vi "Mass Dependent Parameters.vi"(5 "Current Mass Range":i32(ring) items=["Mass Range 1"], 7 "Mass Ranges":T1[](array[typedef]) {"Res" items=["High/High", "Medium/Medium", "Low/Low", "High/Medium", "High/Low", "Medium/High", "Medium/Low", "Low/High", "Low/Medium"]}) -> (3 "Mass Ranges Out":T1[](array[typedef]) {"Res" items=["High/High", "Medium/Medium", "Low/Low", "High/Medium", "High/Low", "Medium/High", "Medium/Low", "Low/High", "Low/Medium"]})   [LabVIEW 2012]
uses:
  Type/_Mass Range Property.ctl
  Type/_Mass Range Parameters.ctl
  Type/_RT Res Type.ctl
  _Global Configuration.vi
panel:
  in  "Current Parameter":u8(ring) items=["Q1-MASS", "Q1-PW", "REFL (FR)", "OR", "MP1-RO (H)", "L7 (G)", "L6 (F)", "Q1-RO", "CC-RO", "Q3-Mass", "Q3-PW", "Q3-RO", "MP2-RO (QO)", "L5 (E)", "L4 (D)", "L3 (C)", "L2 (B)", "L1 (A)"]
  out "Step Value":dbl=1.0 format="%#.3f"
  in  "Stop Value":dbl=1.0 format="%#.3f"
  in  "Start Value":dbl=1.0 format="%#.3f"
  out "# of Parameters":i32=1
  in  "Parameter Table":i32(listbox)
  in  "Delete":bool
  in  "Insert":bool
  out "Dwell Time (ms)":dbl=1.0 format="%#.3f"
  out "Step Mass (amu)":dbl=1.0 format="%#.3f"
  out "Stop Mass (amu)":dbl=1.0 format="%#.3f"
  out "Start Mass (amu)":dbl=1.0 format="%#.3f"
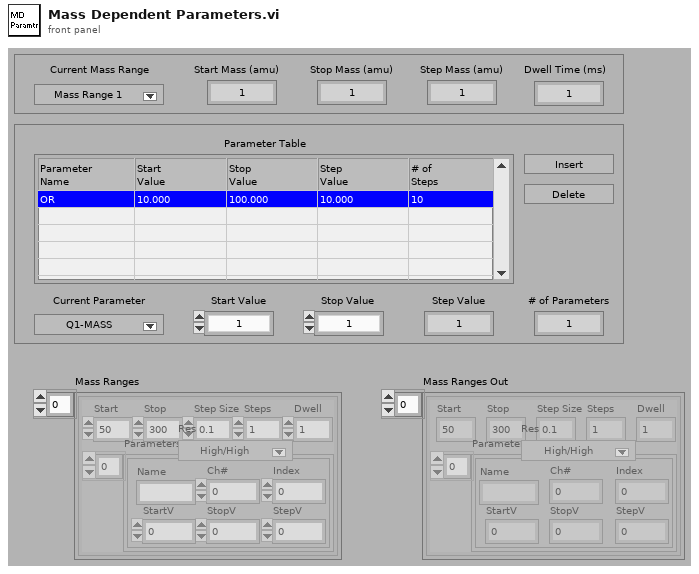
[diagram p1: front panel]
types:
  T1 = typedef "_Mass Range Property.ctl" = cluster{"Start":dbl, "Stop":dbl, "Step Size":dbl, "Steps":i32, "Dwell":dbl, "Parameters":T2[], "Res":T3}
  T2 = typedef "_Mass Range Parameters.ctl" = cluster{"Name":string, "Ch#":u8, "StartV":dbl, "StopV":dbl, "StepV":dbl, "Index":u8}
  T3 = typedef "_RT Res Type.ctl" = u16
  T4 = cluster{"Mass Ranges":T1[], "# of Steps":i32, "Parameters":T2[]}
  T5 = typedef "_RT Instrument 2.ctl" = cluster{"Table":T6[], "Instrument":string[]}
  T6 = typedef "_RT Configuration 2.ctl" = cluster{"Name":string, "Ch#":u8, "Min":dbl, "Max":dbl, "Def+":dbl, "Def-":dbl, "Offset":dbl, "Slope":dbl, "Type":u8, "Description":string, "SettleT":dbl}
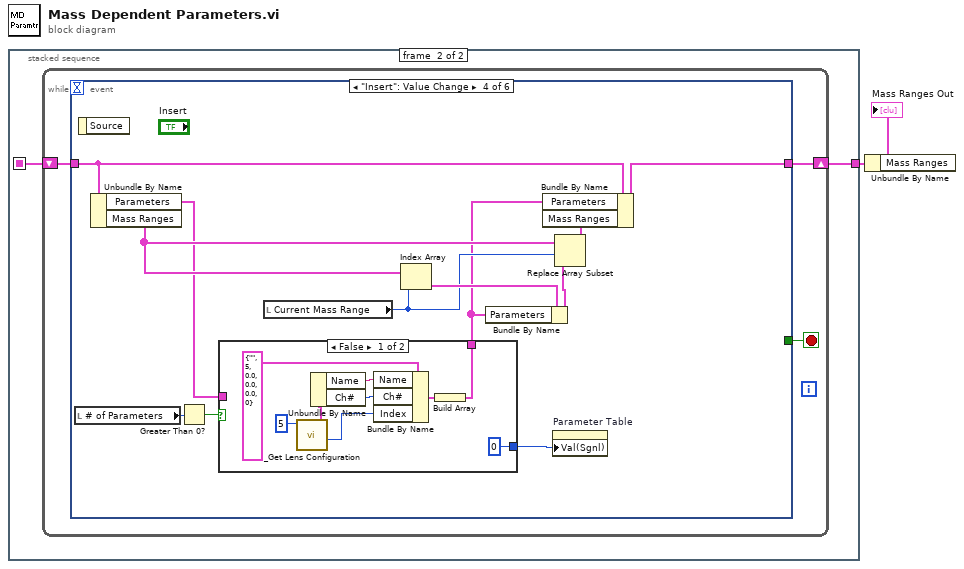
[diagram p0: block diagram]
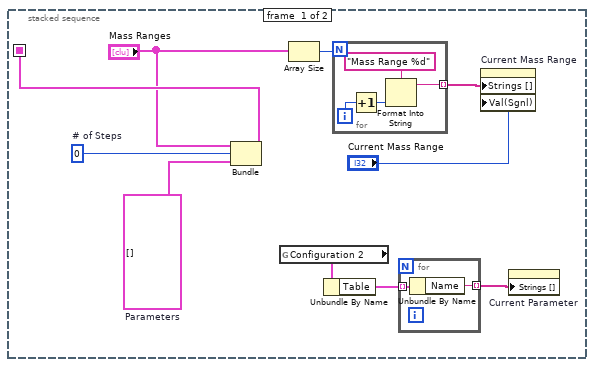
[diagram p2: hidden frame]
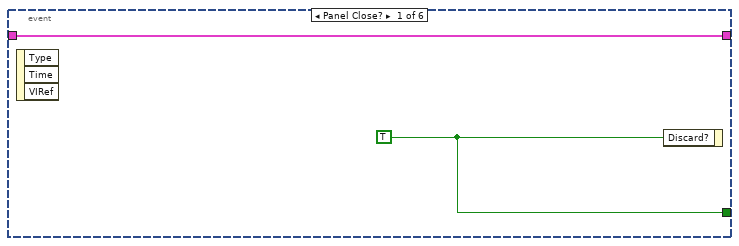
[diagram p3: hidden frame]
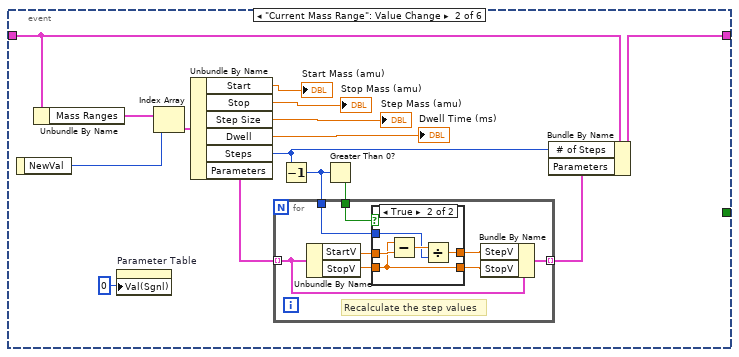
[diagram p4: hidden frame]
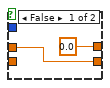
[diagram p5: hidden frame]
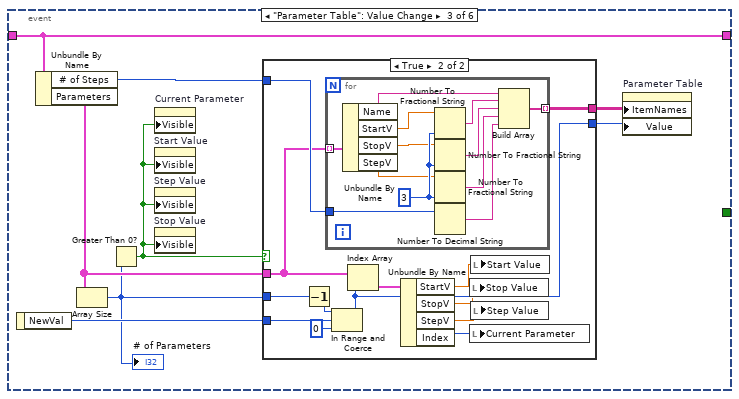
[diagram p6: hidden frame]
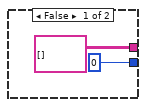
[diagram p7: hidden frame]
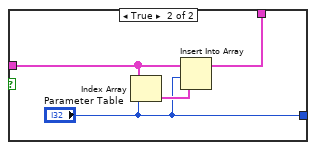
[diagram p8: hidden frame]
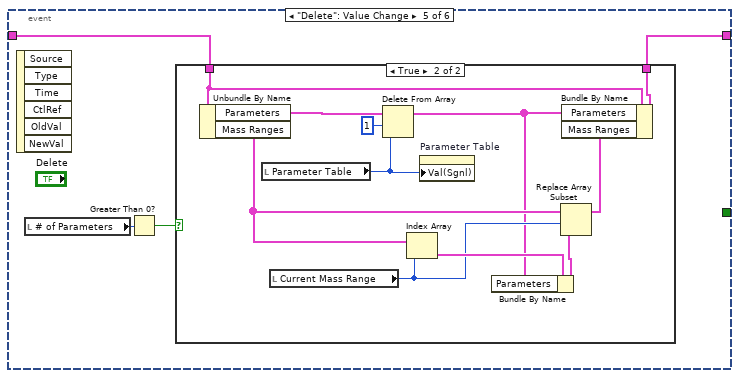
[diagram p9: hidden frame]
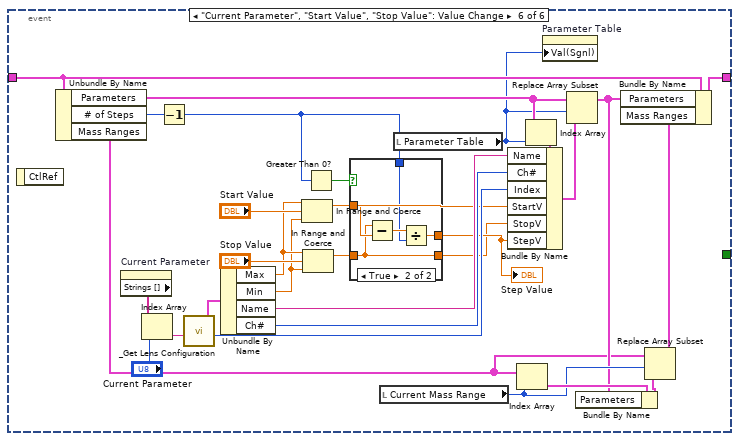
[diagram p11: hidden frame]
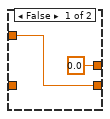
[diagram p12: hidden frame]
diagram:
  n1 = stacked-sequence {
    seq-local: [w5 _] -> [_ w20]
    tunnel: [_ w19] -> w2
    frame #0 {
      w6 = T2[] []  # Parameters
      w7 = 0  # # of Steps
      n2 = Bundle("Mass Ranges"="Mass Ranges", "# of Steps"=w7, "Parameters"=w6) -> (w5:T4)  [unwired: 1 out]
      n3 = global read "_Global Configuration.vi" "Configuration 2"() -> (w11:T5)
      n4 = Array Size(array="Mass Ranges") -> (size(s)=w9:i32)
      n5 = Unbundle By Name(w11) -> ("Table"=w10:T6[])
      n6 = for {
        N: w9 -> [_]
        tunnel: [w13] -> w8 mode=indexing
        i -> [w16]
        n7 = Increment(x=w16) -> (x+1=w14:i32)
        n8 = Format Into String(format string="Mass Range %d", w14) -> (resulting string=w13:string)  [unwired: 2 in, 1 out]
      }
      n9 = for {
        tunnel: w10 -> [w18] mode=indexing
        tunnel: [w17] -> w12 mode=indexing
        n10 = Unbundle By Name(w18) -> ("Name"=w17:string)
      }
      n11 = property on="Current Mass Range" class="Ring (strict)"("Strings []"=w8, "Val(Sgnl)"="Current Mass Range") -> ()  [unwired: 2 in, 2 out]
      n12 = property on="Current Parameter" class="Ring (strict)"("Strings []"=w12) -> ()  [unwired: 2 in, 2 out]
    }
    frame #1 {
      n13 = while {
        shift-right: [w21] -> w19
        shift-left: w20 -> [w22]
        stop <- w23 stop-if-true
        n14 = event shown="[3] \"Insert\": Value Change" {
          selector: _ -> [_ _ _ _ _ _]
          dyn-events: _ -> [_ _ _ _ _ _]
          timeout: _ -> [_ _ _ _ _ _]
          tunnel: [w25 _ _ _ _ _] -> w23
          tunnel: w22 -> [w24 w38 w62 w102 w119 w151]
          tunnel: [w24 w37 w62 w101 w118 w150] -> w21
          event Panel Close? {
            w25 = TRUE ("Discard?")
            n15 = event-data() -> ()  [unwired: 4 out]
            n16 = event-data("Discard?"=w25) -> ()  [unwired: 1 in, 1 out]
          }
          event "Current Mass Range": Value Change {
            n17 = event-data() -> ("NewVal"=w34:i32)  [unwired: 1 out]
            n18 = Unbundle By Name(w38) -> ("Mass Ranges"=w40:T1[])
            n19 = property on="Parameter Table" class="MCListbox (strict)"("Val(Sgnl)"=0 ("Value (Signaling)")) -> ()  [unwired: 2 in, 2 out]
            n20 = Index Array(array=w40, index=w34) -> (element=w39:T1)
            n21 = Unbundle By Name(w39) -> ("Start"=→"Start Mass (amu)":dbl, "Stop"=→"Stop Mass (amu)":dbl, "Step Size"=→"Step Mass (amu)":dbl, "Dwell"=→"Dwell Time (ms)":dbl, "Steps"=w29:i32, "Parameters"=w30:T2[])
            n22 = Decrement(x=w29) -> (x-1=w27:i32)
            n23 = Greater Than 0?(x=w27) -> (x > 0?=w28:bool)
            n24 = for {
              tunnel: w30 -> [w43] mode=indexing
              tunnel: w28 -> [w48]
              tunnel: w27 -> [w45]
              tunnel: [w41] -> w26 mode=indexing
              # "Recalculate the step values"
              n25 = Unbundle By Name(w43) -> ("StartV"=w47:dbl, "StopV"=w46:dbl)
              n26 = case shown="True" w48 {
                tunnel: w46 -> [_ w52]
                tunnel: w47 -> [w49 w54]
                tunnel: [0.0 w53] -> w44
                tunnel: [w49 w52] -> w42
                tunnel: w45 -> [_ w51]
                frame False {
                }
                frame True {
                  n27 = Subtract(x=w52, y=w54) -> (x-y=w55:dbl)
                  n28 = Divide(x=w55, y=w51) -> (x/y=w53:dbl)
                }
              }
              n29 = Bundle By Name(cluster=w43, "StepV"=w44, "StopV"=w42) -> (w41:T2)
            }
            n30 = Bundle By Name(cluster=w38, "# of Steps"=w29, "Parameters"=w26) -> (w37:T4)
          }
          event "Parameter Table": Value Change {
            n31 = event-data() -> ("NewVal"=w63:i32)  [unwired: 1 out]
            n32 = Unbundle By Name(w62) -> ("# of Steps"=w58:i32, "Parameters"=w60:T2[])
            n33 = Array Size(array=w60) -> (size(s)=w57:i32)
            "# of Parameters" <- w57
            n34 = Greater Than 0?(x=w57) -> (x > 0?=w56:bool)
            n35 = property on="Current Parameter" class="Ring (strict)"("Visible"=w56) -> ()  [unwired: 2 in, 2 out]
            n36 = property on="Start Value" class="DigNum (strict)"("Visible"=w56) -> ()  [unwired: 2 in, 2 out]
            n37 = property on="Step Value" class="DigNum (strict)"("Visible"=w56) -> ()  [unwired: 2 in, 2 out]
            n38 = property on="Stop Value" class="DigNum (strict)"("Visible"=w56) -> ()  [unwired: 2 in, 2 out]
            n39 = case shown="True" w56 {
              tunnel: w63 -> [_ w78]
              tunnel: [0 ("lower limit") w75] -> w61
              tunnel: w57 -> [_ w73]
              tunnel: w60 -> [_ w66]
              tunnel: [string[][] [] w68] -> w59
              tunnel: w58 -> [_ w67]
              frame False {
              }
              frame True {
                n40 = Decrement(x=w73) -> (x-1=w77:i32)
                n41 = for {
                  tunnel: w66 -> [w90] mode=indexing
                  tunnel: [w85] -> w68 mode=indexing
                  tunnel: w67 -> [w81]
                  w89 = i16 3 ("precision (6)")
                  n42 = Unbundle By Name(w90) -> ("Name"=w79:string, "StartV"=w86:dbl, "StopV"=w87:dbl, "StepV"=w88:dbl)
                  n43 = Number To Fractional String(number=w86, precision (6)=w89) -> (F-format string=w84:string)  [unwired: 2 out]
                  n44 = Number To Fractional String(number=w87, precision (6)=w89) -> (F-format string=w83:string)  [unwired: 2 out]
                  n45 = Number To Fractional String(number=w88, precision (6)=w89) -> (F-format string=w82:string)  [unwired: 2 out]
                  n46 = Number To Decimal String(number=w81) -> (decimal integer string=w80:string)  [unwired: 1 out]
                  n47 = Build Array(w79, w84, w83, w82, w80) -> (w85:string[])
                }
                n48 = In Range and Coerce(upper limit=w77, x=w78, lower limit=0) -> (coerced(x)=w75:i32)  [unwired: 1 out]
                n49 = Index Array(array=w66, index=w75) -> (element=w74:T2)
                n50 = Unbundle By Name(w74) -> ("StartV"=w69:dbl, "StopV"=w70:dbl, "StepV"=w71:dbl, "Index"=w72:u8)
                n51 = local write "Stop Value"(w70) -> ()
                n52 = local write "Current Parameter"(w72) -> ()
                n53 = local write "Start Value"(w69) -> ()
                n54 = local write "Step Value"(w71) -> ()
              }
            }
            n55 = property on="Parameter Table" class="MCListbox (strict)"("ItemNames"=w59, "Value"=w61) -> ()  [unwired: 2 in, 2 out]
          }
          event "Insert": Value Change {
            n56 = local read "# of Parameters"() -> (w95:i32)
            n57 = event-data() -> ()  [unwired: 2 out]
            n58 = Unbundle By Name(w102) -> ("Parameters"=w93:T2[], "Mass Ranges"=w99:T1[])
            n59 = Greater Than 0?(x=w95) -> (x > 0?=w94:bool)
            n60 = case shown="False" w94 {
              tunnel: w93 -> [_ w114]
              tunnel: [w108 w113] -> w92
              tunnel: [0 ("Parameter Table") "Parameter Table"] -> w91
              frame False {
                n61 = call "_Get Lens Configuration.vi"("Channel #"=u8 5) -> ("Config Row#"=w105:i32, "Lens Configuration"=w107:T6)  [unwired: 1 in, 4 out]
                n62 = Unbundle By Name(w107) -> ("Name"=w103:string, "Ch#"=w104:u8)
                n63 = Bundle By Name(cluster=T2 {"Name"="", "Ch#"=5, "StartV"=0.0, "StopV"=0.0, "StepV"=0.0, "Index"=0}, "Name"=w103, "Ch#"=w104, "Index"=w105) -> (w109:T2)
                n64 = Build Array(w109) -> (w108:T2[])
              }
              frame True {
                n65 = Index Array(array=w114, index="Parameter Table") -> (element=w115:T2)
                n66 = Insert Into Array(array=w114, index="Parameter Table", new element=w115) -> (w113:T2[])
              }
            }
            n67 = local read "Current Mass Range"() -> (w98:i32)
            n68 = Index Array(array=w99, index=w98) -> (element=w100:T1)
            n69 = Bundle By Name(cluster=w100, "Parameters"=w92) -> (w97:T1)
            n70 = property on="Parameter Table" class="MCListbox (strict)"("Val(Sgnl)"=w91) -> ()  [unwired: 2 in, 2 out]
            n71 = Replace Array Subset(array=w99, new element=w97, index=w98) -> (w96:T1[])
            n72 = Bundle By Name(cluster=w102, "Parameters"=w92, "Mass Ranges"=w96) -> (w101:T4)
          }
          event "Delete": Value Change {
            n73 = event-data() -> ()  [unwired: 7 out]
            n74 = local read "# of Parameters"() -> (w116:i32)
            n75 = Greater Than 0?(x=w116) -> (x > 0?=w117:bool)
            n76 = case shown="True" w117 {
              tunnel: w119 -> [w120 w128]
              tunnel: [w120 w127] -> w118
              frame False {
              }
              frame True {
                n77 = Unbundle By Name(w128) -> ("Parameters"=w130:T2[], "Mass Ranges"=w123:T1[])
                n78 = local read "Parameter Table"() -> (w129:i32)
                n79 = local read "Current Mass Range"() -> (w125:i32)
                n80 = Delete From Array(array=w130, length=1, index=w129) -> (array with subset deleted=w122:T2[])  [unwired: 1 out]
                n81 = Index Array(array=w123, index=w125) -> (element=w126:T1)
                n82 = property on="Parameter Table" class="MCListbox (strict)"("Val(Sgnl)"=w129) -> ()  [unwired: 2 in, 2 out]
                n83 = Bundle By Name(cluster=w126, "Parameters"=w122) -> (w124:T1)
                n84 = Replace Array Subset(array=w123, new element=w124, index=w125) -> (w121:T1[])
                n85 = Bundle By Name(cluster=w128, "Parameters"=w122, "Mass Ranges"=w121) -> (w127:T4)
              }
            }
          }
          event "Current Parameter", "Start Value", "Stop Value": Value Change {
            n86 = event-data() -> ()  [unwired: 2 out]
            n87 = Unbundle By Name(w151) -> ("Parameters"=w157:T2[], "# of Steps"=w149:i32, "Mass Ranges"=w136:T1[])
            n88 = property on="Current Parameter" class="Ring (strict)"() -> ("Strings []"=w160:string[])  [unwired: 2 in, 2 out]
            n89 = Index Array(array=w160, index="Current Parameter") -> (element=w161:string)
            n90 = Decrement(x=w149) -> (x-1=w133:i32)
            n91 = call "_Get Lens Configuration.vi"("Name"=w161) -> ("Config Row#"=w152:i32, "Lens Configuration"=w159:T6)  [unwired: 1 in, 4 out]
            n92 = Unbundle By Name(w159) -> ("Max"=w146:dbl, "Min"=w145:dbl, "Name"=w155:string, "Ch#"=w153:u8)
            n93 = In Range and Coerce(upper limit=w146, x="Start Value", lower limit=w145) -> (coerced(x)=w143:dbl)  [unwired: 1 out]
            n94 = In Range and Coerce(upper limit=w146, x="Stop Value", lower limit=w145) -> (coerced(x)=w144:dbl)  [unwired: 1 out]
            n95 = Greater Than 0?(x=w133) -> (x > 0?=w134:bool)
            n96 = case shown="True" w134 {
              tunnel: w144 -> [_ w164]
              tunnel: w143 -> [w162 w167]
              tunnel: w133 -> [_ w166]
              tunnel: [0.0 w165] -> w142
              tunnel: [w162 w164] -> w132
              frame False {
              }
              frame True {
                n97 = Subtract(x=w164, y=w167) -> (x-y=w168:dbl)
                n98 = Divide(x=w168, y=w166) -> (x/y=w165:dbl)
              }
            }
            "Step Value" <- w142
            n99 = local read "Current Mass Range"() -> (w139:i32)
            n100 = local read "Parameter Table"() -> (w141:i32)
            n101 = Index Array(array=w136, index=w139) -> (element=w140:T1)
            n102 = Index Array(array=w157, index=w141) -> (element=w156:T2)
            n103 = Bundle By Name(cluster=w156, "Name"=w155, "Ch#"=w153, "Index"=w152, "StartV"=w143, "StopV"=w132, "StepV"=w142) -> (w154:T2)
            n104 = property on="Parameter Table" class="MCListbox (strict)"("Val(Sgnl)"=w141) -> ()  [unwired: 2 in, 2 out]
            n105 = Replace Array Subset(array=w157, new element=w154, index=w141) -> (w137:T2[])
            n106 = Bundle By Name(cluster=w140, "Parameters"=w137) -> (w138:T1)
            n107 = Replace Array Subset(array=w136, new element=w138, index=w139) -> (w135:T1[])
            n108 = Bundle By Name(cluster=w151, "Parameters"=w137, "Mass Ranges"=w135) -> (w150:T4)
          }
        }
      }
    }
  }
  n109 = Unbundle By Name(w2) -> ("Mass Ranges"=→"Mass Ranges Out":T1[])
